vi "Error_handling.vi"(8 "Error In":errorcluster, 11 "User Event in":refnum<user-event>) -> (0 "Error Out":errorcluster, 3 "User Event out":refnum<user-event>)   [LabVIEW 2021, in "Main.lvlib" / "Main_Programs_SubVIs.lvlib"]
doc: "This subVI is used to detect and generate ERROR user event so all the while loops are stopped."
uses:
  Main_Programs_SubVIs.lvlib
  <vilib>/Utility/error.llb/DialogType.ctl
  <vilib>/event_ctls.llb/usereventprio.ctl
panel:
  # "Input"
  # "Output"
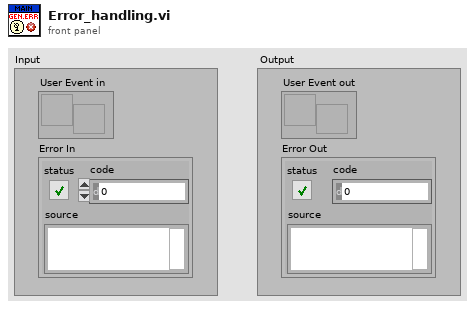
[diagram p1: front panel]
types:
  T1 = typedef "usereventprio.ctl" = enum32{"high priority", "normal priority"}
  T2 = typedef "DialogType.ctl" = u16
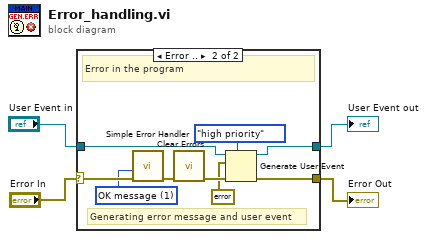
[diagram p0: block diagram]
diagram:
  n1 = case shown="Error .." "Error In" {
    selector: "Error In" -> [w5 w11]
    tunnel: "User Event in" -> [w6 w15]
    tunnel: [w6 w14] -> w2
    tunnel: [w5 w13] -> w1
    frame No Error {
      # "There is no error in the program"
    }
    frame Error {
      w10 = T2 1 items=["no dialog", "OK message", "continue or stop message", "OK message + warnings", "continue/stop + warnings"] ("type of dialog (OK msg:1)")
      # "Generating error message and user event"
      # "Error in the program"
      n2 = call <vilib>:"Simple Error Handler.vi"("type of dialog (OK msg:1)"=w10, "error in (no error)"=w11) -> ("error out"=w12:errorcluster)  [unwired: 3 in, 4 out]
      n3 = call <vilib>:"Clear Errors.vi"("error in (no error)"=w12) -> ("error out"=w9:errorcluster)  [unwired: 5 in, 1 out]
      n4 = Generate User Event(priority (normal)=usereventprio."high priority", user event=w15, event data cluster=errorcluster {"status"=FALSE, "code"=0, "source"=""} ("event data"), error in=w9) -> (user event out=w14:refnum<user-event>, error out=w13:errorcluster)
    }
  }
  "User Event out" <- w2
  "Error Out" <- w1
